vi "_Manager.vi"(7 "Action":T1, 8 "Error In":errorcluster, 11 "Set Value":variant) -> (0 "Error Out":errorcluster)   [LabVIEW 2015, in "Logger.lvlib" / "File.lvlib"]
uses:
  File.lvlib
  _Action.ctl
  Public/Controls/Message.ctl
  Public/Controls/Tag.ctl
  _Create ISO 8601 File Name.vi
  _Write Header.vi
  _Create Calendar Folder Tree.vi
  _Get Oldest File.vi
  Public/Utility/Create Message CSV.vi
  _Create Level String.vi
  _Strip Whitespace.vi
  <vilib>/dlg_ctls.llb/Space Constant.vi
  <vilib>/Utility/libraryn.llb/Check if File or Folder Exists.vi
  Logger.lvlib
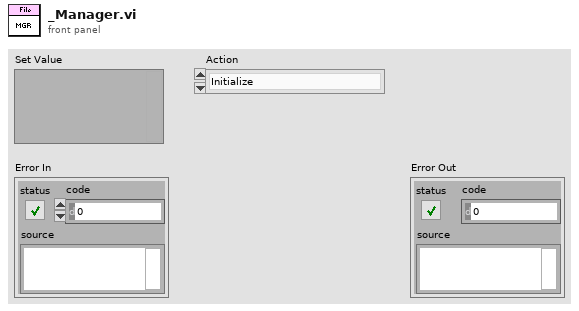
[diagram p1: front panel]
types:
  T1 = typedef "Logger.lvlib/File.lvlib/_Action.ctl" = enum16{"Initialize", "Set Maximum File Size", "Set Maximum File Count", "Set Root Folder", "Set Enable Calendar Folder Tree", "Set File Extension", "Start", "Write", "Stop", "Shutdown"}
  T2 = typedef "Logger.lvlib/Message.ctl" = cluster{"Time Stamp":timestamp, "Tag":T3, "Source":string, "Text":string}
  T3 = typedef "Logger.lvlib/Tag.ctl" = enum16{"Fatal", "Error", "Warn", "Info", "Debug", "Trace"}
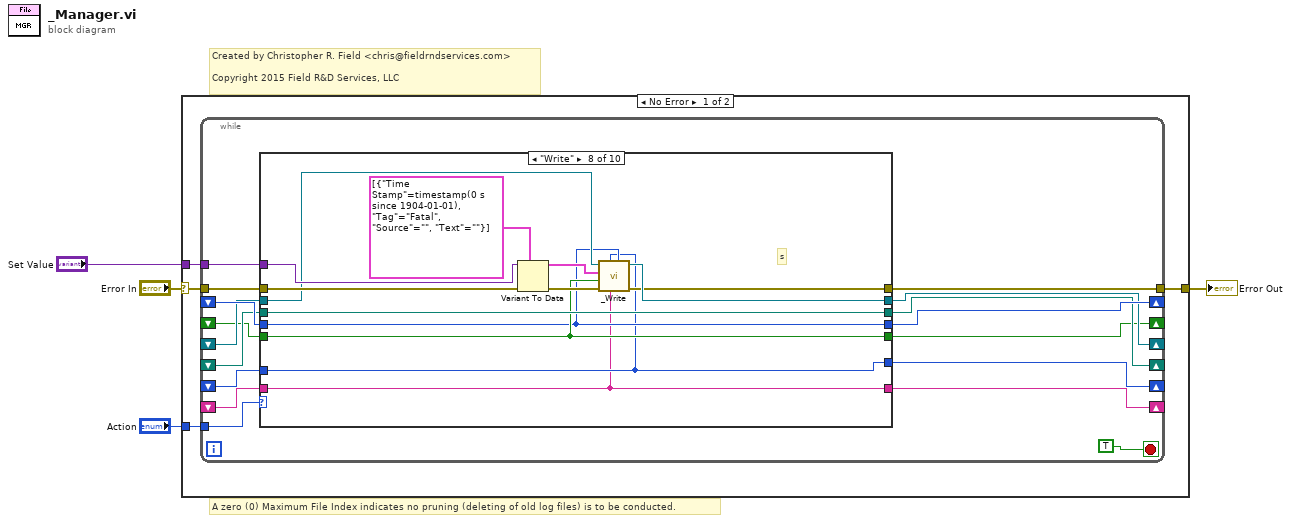
[diagram p0: block diagram]
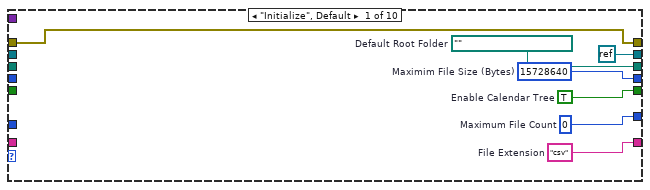
[diagram p2: hidden frame]
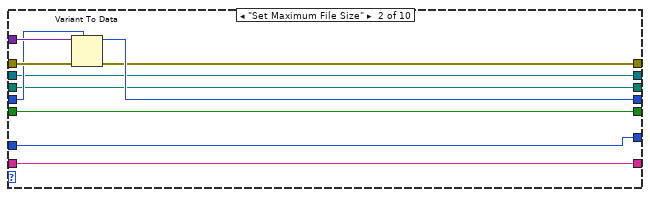
[diagram p3: hidden frame]
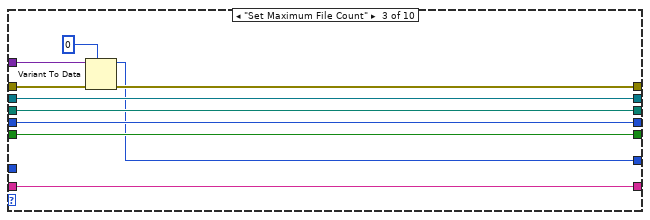
[diagram p4: hidden frame]
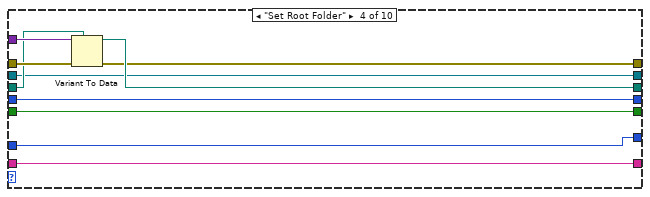
[diagram p5: hidden frame]
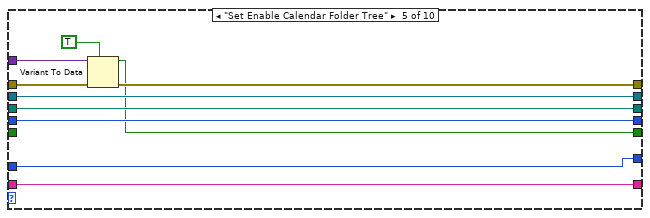
[diagram p6: hidden frame]
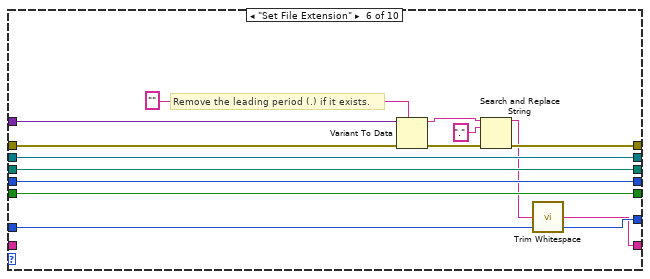
[diagram p7: hidden frame]
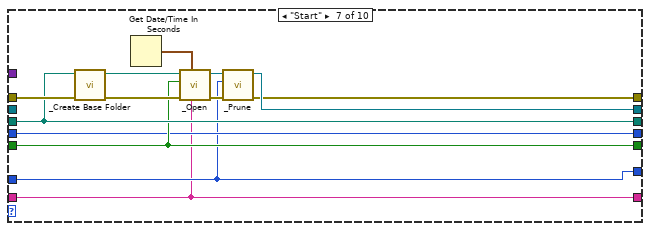
[diagram p8: hidden frame]
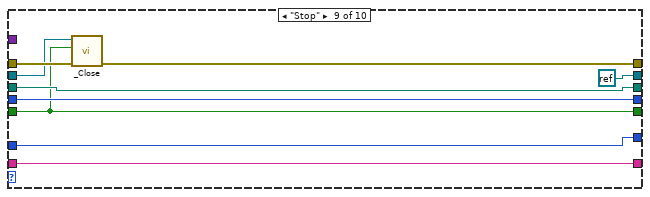
[diagram p9: hidden frame]
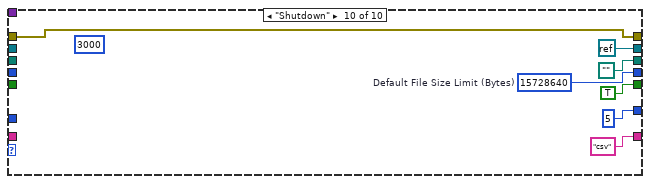
[diagram p10: hidden frame]
diagram:
  # "A zero (0) Maximum File Index indicates no pruning (deleting of old log files) is to be conducted."
  # "Created by Christopher R. Field <chris@fieldrndservices.com>\n\nCopyright 2015 Field R&D Services, LLC"
  n1 = case shown="No Error" "Error In" {
    selector: "Error In" -> [w7 w129]
    tunnel: "Action" -> [w8 _]
    tunnel: "Set Value" -> [w6 _]
    tunnel: [w5 w129] -> w1
    frame No Error {
      n2 = while {
        tunnel: w8 -> [w24]
        shift-right: [w23] -> _
        shift-left: _ -> [w18]
        shift-right: [w22] -> _
        shift-left: _ -> [w15]
        shift-right: [w21] -> _
        shift-left: _ -> [w16]
        tunnel: w7 -> [w20]
        tunnel: w6 -> [w19]
        tunnel: [w17] -> w5
        shift-right: [w14] -> _
        shift-left: _ -> [w13]
        shift-right: [w12] -> _
        shift-left: _ -> [w11]
        shift-right: [w10] -> _
        shift-left: _ -> [w9]
        stop <- TRUE stop-if-true
        n3 = case shown="\"Write\"" w24 {
          tunnel: [w32 w39 w46 w62 w72 w86 w89 w102 w117 w125] -> w23
          tunnel: [refnum<k0> refnum w36 w48 w56 w68 w83 w92 w105 refnum<k0> refnum refnum<k0> refnum] -> w22
          tunnel: [w30 w37 w49 w58 w67 w82 w96 w109 w118 path ""] -> w21
          tunnel: w20 -> [w29 w42 w52 w60 w70 w84 w97 w111 w121 w127]
          tunnel: w19 -> [_ w41 w51 w61 w71 w85 _ w112 _ _]
          tunnel: w18 -> [_ w40 w46 w62 w72 w86 w89 w102 w117 _]
          tunnel: [w29 w38 w50 w57 w69 w77 w90 w104 w116 w127] -> w17
          tunnel: w16 -> [_ w37 w49 w59 w67 w82 w96 w109 w118 _]
          tunnel: w15 -> [_ w36 w48 w56 w68 w83 _ w106 w120 _]
          tunnel: [w28 w35 w47 w55 w65 w79 w93 w103 w114 TRUE] -> w14
          tunnel: w13 -> [_ w35 w47 w55 _ w79 w93 w103 w114 _]
          tunnel: [w27 w34 w44 w54 w64 w81 w88 w101 w115 5] -> w12
          tunnel: w11 -> [_ w34 _ w54 w64 w81 w88 w101 w115 _]
          tunnel: [w26 w33 w43 w53 w63 w73 w87 w100 w113 "csv"] -> w10
          tunnel: w9 -> [_ w33 w43 w53 w63 _ w87 w100 w113 _]
          frame "Initialize", Default {
            w26 = "csv"  # File Extension
            w27 = 0  # Maximum File Count
            w28 = TRUE  # Enable Calendar Tree
            w30 = path ""  # Default Root Folder
            w32 = i64 15728640  # Maximim File Size (Bytes)
          }
          frame "Set Maximum File Size" {
            n4 = Variant To Data(error in=w42, type=w40, Variant=w41) -> (data=w39:i64, error out=w38:errorcluster)
          }
          frame "Set Maximum File Count" {
            n5 = Variant To Data(error in=w52, type=0, Variant=w51) -> (data=w44:i32, error out=w50:errorcluster)
          }
          frame "Set Root Folder" {
            n6 = Variant To Data(error in=w60, type=w59, Variant=w61) -> (data=w58:path, error out=w57:errorcluster)
          }
          frame "Set Enable Calendar Folder Tree" {
            n7 = Variant To Data(error in=w70, type=TRUE, Variant=w71) -> (data=w65:bool, error out=w69:errorcluster)
          }
          frame "Set File Extension" {
            # "Remove the leading period (.) if it exists."
            n8 = Variant To Data(error in=w84, type="", Variant=w85) -> (data=w76:string, error out=w78:errorcluster)
            n9 = Search and Replace String(input string=w76, search string=".", error in=w78) -> (result string=w74:string, error out=w77:errorcluster)  [unwired: 5 in, 2 out]
            n10 = call <vilib>:"Trim Whitespace.vi"("string"=w74) -> ("trimmed string"=w73:string)  [unwired: 1 in]
          }
          frame "Start" {
            n11 = call "_Create Base Folder.vi"("Error In"=w97, "Root Folder"=w96) -> ("Error Out"=w98:errorcluster, "Base Folder"=w99:path)  [unwired: 8 in]
            n12 = Get Date/Time In Seconds() -> (seconds since 1Jan1904=w94:timestamp)
            n13 = call "_Open.vi"("File Extension"=w87, "Start Time Stamp"=w94, "Error In"=w98, "Enable Calendar Tree"=w93, "Base Folder"=w99) -> ("Error Out"=w91:errorcluster, "Log Out"=w95:refnum<file>)  [unwired: 5 in]
            n14 = call "_Prune.vi"("Error In"=w91, "Maximum File Count"=w88, "File In"=w95) -> ("Error Out"=w90:errorcluster, "File Out"=w92:refnum<file>)  [unwired: 7 in]
          }
          frame "Write" {
            # "s"
            n15 = Variant To Data(error in=w111, type=T2[] [{"Time Stamp"=timestamp(0 s since 1904-01-01), "Tag"=enum."Fatal", "Source"="", "Text"=""}], Variant=w112) -> (data=w108:T2[], error out=w107:errorcluster)
            n16 = call "_Write.vi"("Maximum File Size (Bytes)"=w102, "File Extension"=w100, "Maximum File Count"=w101, "Error In"=w107, "Enable Calendar Tree"=w103, "Messages"=w108, "Log In"=w106) -> ("Error Out"=w104:errorcluster, "Log Out"=w105:refnum<file>)  [unwired: 3 in]
          }
          frame "Stop" {
            n17 = call "_Close.vi"("Error In"=w121, "Enable Calendar Tree"=w114, "Log In"=w120) -> ("Error Out"=w116:errorcluster)  [unwired: 7 in, 1 out]
          }
          frame "Shutdown" {
            (unwired) 3000 ("Write Period (ms)")
            w125 = i64 15728640  # Default File Size Limit (Bytes)
          }
        }
      }
    }
    frame Error {
    }
  }
  "Error Out" <- w1
